vi "Xml_Load_Voltages.vi"(7 "Version String":string, 8 "error in (no error)":errorcluster, 10 "XML Path":path=path "D:/TEST.xml", 11 "Refnum Clust":refnum<vi>) -> (0 "error out":errorcluster)   [LabVIEW 2017]
uses:
  controls/VOLTAGES_Inputs.ctl
  controls/HEXA_Inputs.ctl
  controls/QUAD_Inputs.ctl
panel:
  in  "VOLTAGES Inputs":T1={"Hexa 1"={"Used"=TRUE, "Voltage"=25.0}, "Hexa 2"={"Used"=TRUE, "Voltage"=25.0}, "Hexa 3"={"Used"=TRUE, "Voltage"=25.0}, "Quad 1"={"Used"=TRUE, "Voltage"=25.0}, "Quad 2"={"Used"=TRUE, "Voltage"=25.0}, "Quad 3"={"Used"=TRUE, "Voltage"=25.0}}
  # "HEXAPOLE"
  # "QUADRIPOLE"
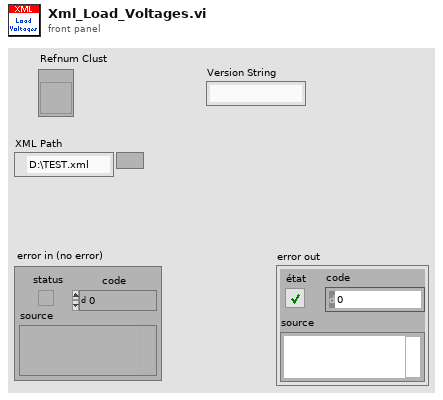
[diagram p1: front panel]
types:
  T1 = typedef "VOLTAGES_Inputs.ctl" = cluster{"Hexa 1":T2, "Hexa 2":T2, "Hexa 3":T2, "Quad 1":T3, "Quad 2":T3, "Quad 3":T3}
  T2 = typedef "HEXA_Inputs.ctl" = cluster{"Used":bool, "Voltage":dbl}
  T3 = typedef "QUAD_Inputs.ctl" = cluster{"Used":bool, "Voltage":dbl}
  T4 = cluster{"Hexa 1":T2, "Hexa 2":T2, "Hexa 3":T2, "Quad 1":T3, "Quad 2":T3, "Quad 3":T3}
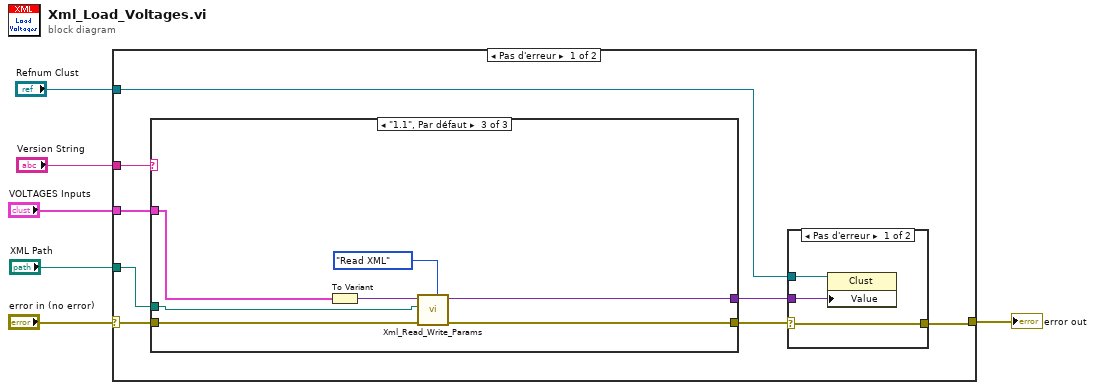
[diagram p0: block diagram]
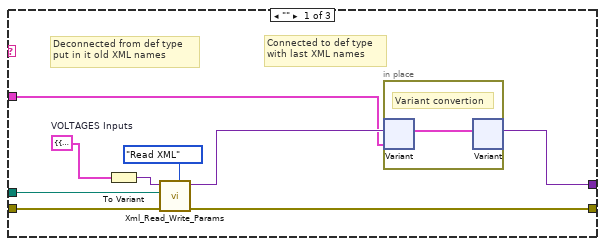
[diagram p3: hidden frame]
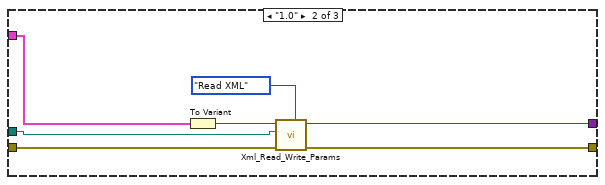
[diagram p4: hidden frame]
diagram:
  n1 = case shown="Pas d'erreur" "error in (no error)" {
    selector: "error in (no error)" -> [w14 w43]
    tunnel: [w9 w43] -> w6
    tunnel: "XML Path" -> [w13 _]
    tunnel: "Version String" -> [w12 _]
    tunnel: "Refnum Clust" -> [w7 _]
    tunnel: "VOLTAGES Inputs" -> [w11 _]
    frame No Error {
      n2 = case shown="\"1.1\", Par défaut" w12 {
        tunnel: w14 -> [w25 w33 w40]
        tunnel: [w21 w31 w38] -> w10
        tunnel: [w23 w32 w39] -> w8
        tunnel: w13 -> [w22 w30 w37]
        tunnel: w11 -> [w19 w29 w36]
        frame "" {
          w20 = T4 {"Hexa 1"={"Used"=TRUE, "Voltage"=25.0}, "Hexa 2"={"Used"=TRUE, "Voltage"=25.0}, "Hexa 3"={"Used"=TRUE, "Voltage"=25.0}, "Quad 1"={"Used"=TRUE, "Voltage"=25.0}, "Quad 2"={"Used"=TRUE, "Voltage"=25.0}, "Quad 3"={"Used"=TRUE, "Voltage"=25.0}}  # VOLTAGES Inputs
          # "Connected to def type\nwith last XML names"
          # "Deconnected from def type\nput in it old XML names"
          n3 = To Variant(anything=w20) -> (Variant=w26:variant)
          n4 = call "Xml_Read_Write_Params.vi"("Variant"=w26, "XML Path"=w22, "error in (no error)"=w25, "Command"=enum16{"Read XML", "Set", "Get", "Write XML"}."Read XML") -> ("Variant Output"=w24:variant, "error out"=w21:errorcluster)  [unwired: 3 in, 1 out]
          n5 = in-place "Structure Élément en place" {
            # "Variant convertion"
            n6 = in-place-variant #1(w24, w19) -> (w28:T1)  [unwired: 1 out]
            n7 = in-place-variant #1(w28) -> (w23:variant)  [unwired: 1 out]
          }
        }
        frame "1.0" {
          n8 = To Variant(anything=w29) -> (Variant=w34:variant)
          n9 = call "Xml_Read_Write_Params.vi"("Variant"=w34, "XML Path"=w30, "error in (no error)"=w33, "Command"=enum16{"Read XML", "Set", "Get", "Write XML"}."Read XML") -> ("Variant Output"=w32:variant, "error out"=w31:errorcluster)  [unwired: 3 in, 1 out]
        }
        frame "1.1", Default {
          n10 = To Variant(anything=w36) -> (Variant=w41:variant)
          n11 = call "Xml_Read_Write_Params.vi"("Variant"=w41, "XML Path"=w37, "error in (no error)"=w40, "Command"=enum16{"Read XML", "Set", "Get", "Write XML"}."Read XML") -> ("Variant Output"=w39:variant, "error out"=w38:errorcluster)  [unwired: 3 in, 1 out]
        }
      }
      n12 = case shown="Pas d'erreur" w10 {
        selector: w10 -> [w16 w18]
        tunnel: w7 -> [w17 _]
        tunnel: [w16 w18] -> w9
        tunnel: w8 -> [w15 _]
        frame No Error {
          n13 = property class="Clust"(reference=w17, "Value"=w15) -> ()  [unwired: 1 in, 2 out]
        }
        frame Error {
        }
      }
    }
    frame Error {
    }
  }
  "error out" <- w6
